vi "Execute.vi"(8 "error in":errorcluster, 11 "DBL STEP in":refnum<class "DBL STEP.lvclass">) -> (0 "error out":errorcluster, 1 "Next Step?":bool, 2 "MSG":string, 3 "DBL STEP out":refnum<class "DBL STEP.lvclass">)   [LabVIEW 2014, in "DBL STEP.lvlib" / "DBL STEP.lvclass"]
uses:
  DBL STEP.lvclass
  Send MSG STEP.lvlibp/Send MSG STEP.lvclass
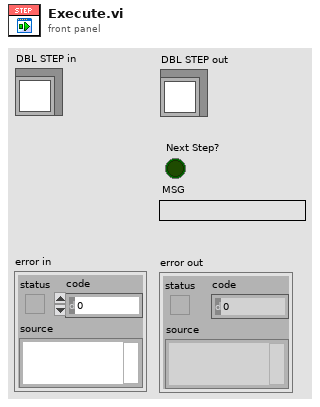
[diagram p1: front panel]
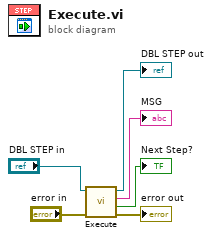
[diagram p0: block diagram]
diagram:
  n1 = call-parent "Execute.vi"("error in"="error in", "STEP in"="DBL STEP in") -> ("error out"=→"error out":errorcluster, "Next Step?"=→"Next Step?":bool, "MSG"=→"MSG":string, "STEP out"=→"DBL STEP out":refnum<class "DBL STEP.lvclass">)  [unwired: 6 in]
